vi "Filter Excel Data.vi"(8 "error in (no error)":errorcluster, 9 "Row":cluster{"Row index":i32, "Length":i32}={"Row index"=0, "Length"=2}, 10 "Column":cluster{"Col index":i32, "Length":i32}={"Col index"=0, "Length"=2}, 11 "2D Data In":string[][](array[string])) -> (0 "error out":errorcluster, 3 "2D Data Out":string[][](array[string]))   [LabVIEW 2016, in "User Interface.lvlib"]
uses:
  User Interface.lvlib
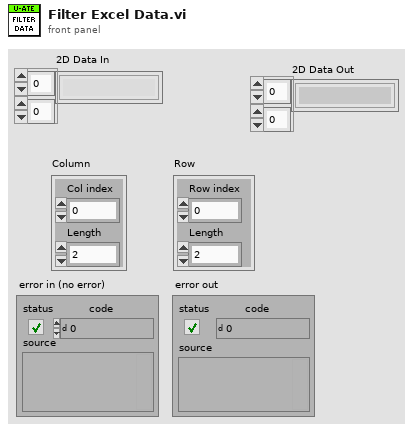
[diagram p1: front panel]
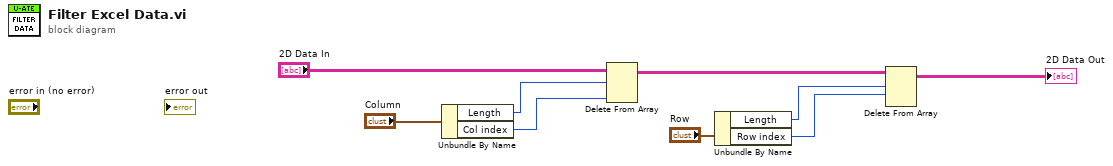
[diagram p0: block diagram]
diagram:
  n1 = Unbundle By Name("Column") -> ("Length"=w4:i32, "Col index"=w5:i32)
  n2 = Delete From Array(array="2D Data In", length=w4, index (col)=w5) -> (array with subset deleted=w9:string[][])  [unwired: 1 in, 1 out]
  n3 = Unbundle By Name("Row") -> ("Length"=w1:i32, "Row index"=w2:i32)
  n4 = Delete From Array(array=w9, length=w1, index (row)=w2) -> (array with subset deleted=→"2D Data Out":string[][])  [unwired: 1 in, 1 out]
